vi "SigInfo LoadFromMZInfoFile.vi"(8 "error in (no error)":errorcluster) -> (0 "error out":errorcluster, 3 "mzInfo out":refnum<class "SigInfo.lvclass">)   [LabVIEW 2018, in "SigInfo.lvclass"]
uses:
  SigInfo.lvclass
  SigInfo.lvclass/SigInfo.ctl
  <userlib>/_OpenG.lib/file/file.llb/File Exists - Scalar__ogtk.vi
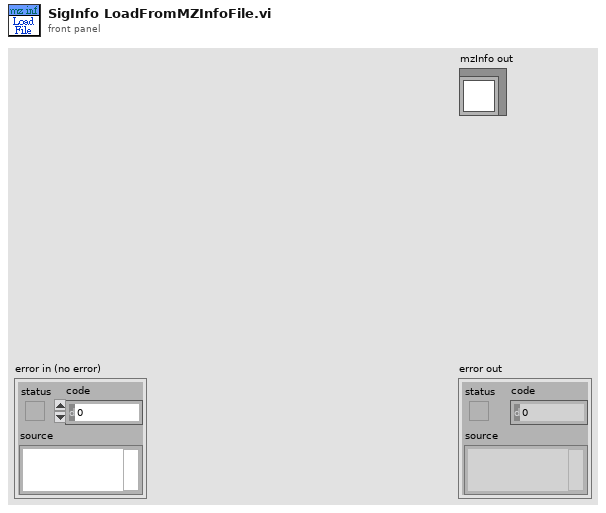
[diagram p1: front panel]
types:
  T1 = enum16{"open", "replace", "create", "open or create", "replace or create", "replace or create with confirmation"}
  T2 = cluster{"mzID":u64, "SignalInfo":cluster{"Label":string, "dt":dbl, "Length":u32, "RefVolt":dbl, "mzTable":cluster{"t":dbl[], "mz":dbl[], "beta":dbl[]}}[]}
  T3 = typedef "Semaphore RefNum" = refnum<k1>
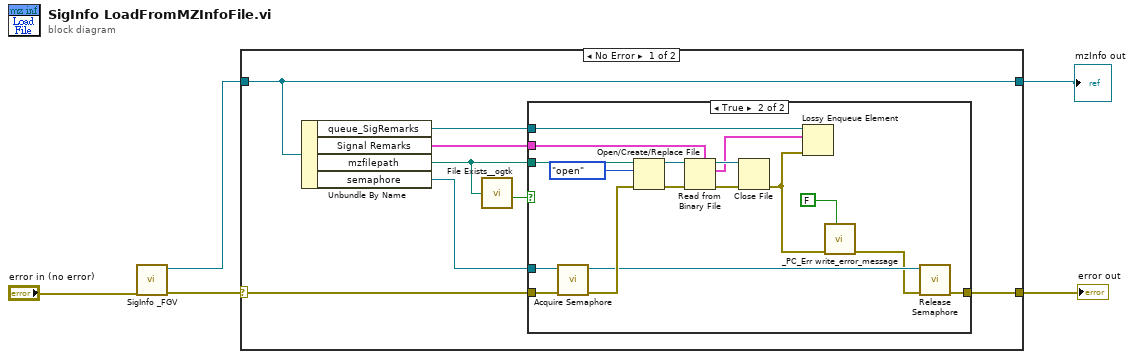
[diagram p0: block diagram]
diagram:
  n1 = call "SigInfo _FGV.vi"("error in (no error)"="error in (no error)") -> ("error out"=w1:errorcluster, "mzInfo out"=w2:refnum<class "SigInfo.lvclass">)  [unwired: 9 in]
  n2 = case shown="No Error" w1 {
    selector: w1 -> [w8 w33]
    tunnel: [w6 w33] -> w5
    tunnel: [w11 w32] -> w4
    tunnel: w2 -> [w11 w32]
    frame No Error {
      n3 = Unbundle By Name(w11) -> ("queue_SigRemarks"=w12:refnum<queue>, "Signal Remarks"=w13:T2, "mzfilepath"=w10:path, "semaphore"=w7:T3)
      n4 = call-poly <userlib>:"File Exists__ogtk.vi"("file path"=w10) -> ("exists"=w9:bool)  [unwired: 6 in, 1 out]
      n5 = case shown="True" w9 {
        tunnel: w13 -> [_ w31]
        tunnel: w12 -> [_ w28]
        tunnel: w10 -> [_ w23]
        tunnel: w8 -> [w14 w22]
        tunnel: w7 -> [_ w21]
        tunnel: [w14 w18] -> w6
        frame False {
        }
        frame True {
          n6 = call <vilib>:"Acquire Semaphore.vi"("error in (no error)"=w22, "semaphore"=w21) -> ("error out"=w20:errorcluster, "semaphore out"=w19:T3)  [unwired: 3 in, 1 out]
          n7 = Open/Create/Replace File(file path (use dialog)=w23, error in=w20, operation (0:open)=T1."open") -> (refnum out=w24:refnum<file>, error out=w26:errorcluster)  [unwired: 3 in, 1 out]
          n8 = Read from Binary File(5:w31, 8:w26, 11:w24) -> (0:w30:errorcluster, 2:w27:T2, 3:w29:refnum<file>)  [unwired: 3 in, 1 out]
          n9 = Close File(refnum=w29, error in=w30) -> (error out=w17:errorcluster)  [unwired: 1 out]
          n10 = Lossy Enqueue Element(queue=w28, element=w27, error in (no error)=w17) -> ()  [unwired: 4 out]
          n11 = call "_PC_Err write_error_message.vi"("show msg( T )"=FALSE, "error in"=w17) -> ("error out"=w16:errorcluster)  [unwired: 9 in]
          n12 = call <vilib>:"Release Semaphore.vi"("error in (no error)"=w16, "semaphore"=w19) -> ("error out"=w18:errorcluster)  [unwired: 4 in, 1 out]
        }
      }
    }
    frame Error {
    }
  }
  "error out" <- w5
  "mzInfo out" <- w4
